vi "Main.vi"(8 "error in (no error)":errorcluster, 11 "ModuleAdmin":refnum<class "ModuleAdmin.lvclass">) -> ()   [LabVIEW 2014, in "SpecAnModule.lvlib"]
uses:
  SpecAnModule.lvlib
  <userlib>/NIST/ModuleAdminLib/ModuleAdmin/ModuleAdmin.lvclass
  SpecAnPlugins/SpecAnBaseClass/SpecAnBase.lvclass
  PublicAPI/Arguments/Requests/clStopArgument.ctl
  <userlib>/NIST/ModuleAdminLib/ModuleAdmin/ModuleAdmin.lvclass/ModuleAdmin.ctl
  <userlib>/NIST/BaseClasses/BasePlugin_class/BasePlugin.lvclass/BasePlugin.ctl
  <vilib>/Utility/error.llb/DialogType.ctl
  <userlib>/NIST/ModuleAdminLib/ModuleAdmin/Accessors/Read ShowPanel_.vi
  <userlib>/NIST/ModuleAdminLib/ModuleAdmin/Accessors/Write ShowPanel_.vi
  <userlib>/NIST/BaseClasses/BasePlugin_class/Accessors/Write PluginIniFilePath.vi
  <userlib>/NIST/BaseClasses/BasePlugin_class/Accessors/Read PluginIniFilePath.vi
  <userlib>/NIST/ModuleAdminLib/ModuleAdmin/Accessors/Read CloneRegRef.vi
  <vilib>/Utility/error.llb/Error Cluster From Error Code.vi
  <vilib>/ErrorRing/Error Ring.xnode
  <userlib>/NIST/ModuleAdminLib/CloneRegistration/CloneRegistration.lvclass
  <userlib>/NIST/BaseClasses/Object_class/BaseObject.lvclass
  <userlib>/NIST/ModuleAdminLib/ModuleAdmin.lvlib
panel:
  out "error out":errorcluster
  # "This is the template for your cloneable module.\nYou should modifiy this to perform the functionality\nthat you want it to perform"
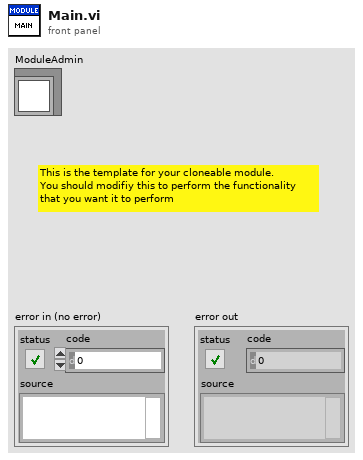
[diagram p1: front panel]
types:
  T1 = typedef "SpecAnModule.lvlib/clRequestEvents.ctl" = cluster{"StopRequest":refnum<user-event>, "PathToINI":refnum<user-event>, " LoadPlugin":refnum<user-event>, "ShowPanel":refnum<user-event>, "PrefDlg":refnum<user-event>, "Initialize":refnum<user-event>, "Close":refnum<user-event>, "Abort":refnum<user-event>, "Fetch":refnum<user-event>, "Read":refnum<user-event>, "Configure":refnum<user-event>, "GetTraceName":refnum<user-event>, "Initiate":refnum<user-event>}
  T2 = typedef "SpecAnModule.lvlib/clBroadcastEvents.ctl" = cluster{"DidInit":refnum<user-event>, "StatusUpdate":refnum<user-event>, "ErrorReport":refnum<user-event>, "DidStop":refnum<user-event>, "PathToINI":refnum<user-event>, "TraceName":refnum<user-event>}
  T3 = typedef "SpecAnModule.lvlib/clStopArgument.ctl" = cluster{"Exit via Stop Module Req?":bool, "Wait for Module to stop?":bool, "ModuleAdmin":refnum<class "ModuleAdmin.lvclass">}
  T4 = enum32{"Invalid", "Standard", "Closed", "Hidden", "Minimized", "Maximized"}
  T5 = typedef "DialogType.ctl" = u16
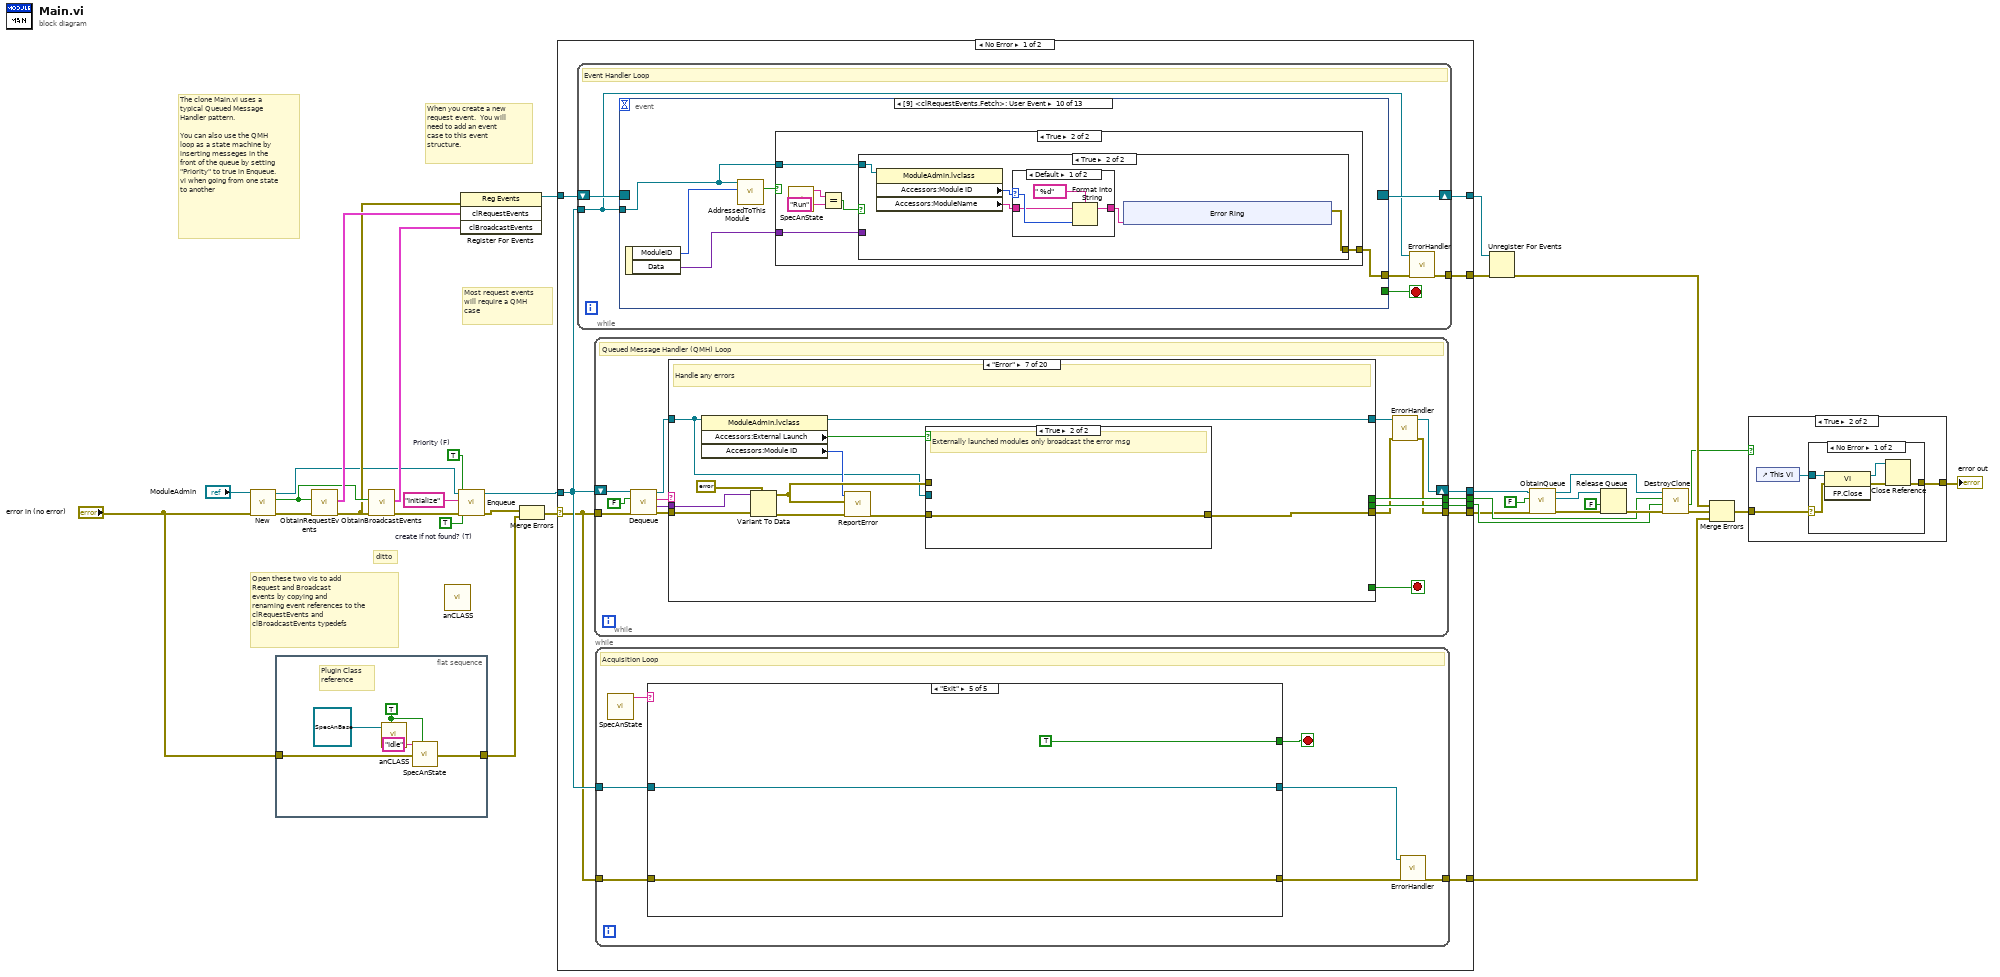
[diagram p0: block diagram]
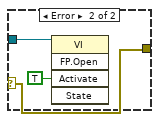
[diagram p3: hidden frame]
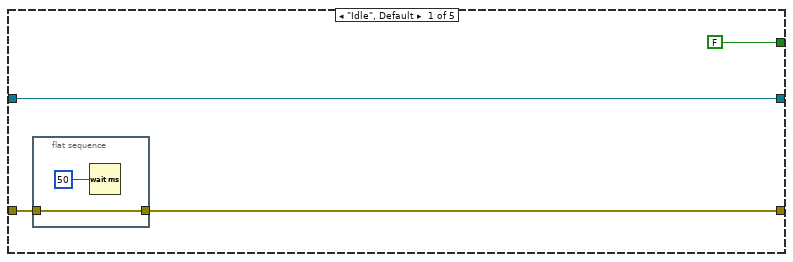
[diagram p4: hidden frame]
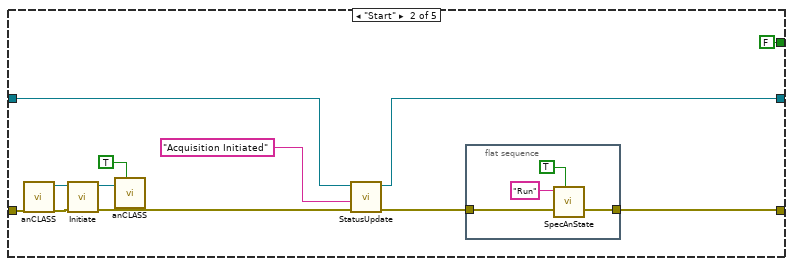
[diagram p5: hidden frame]
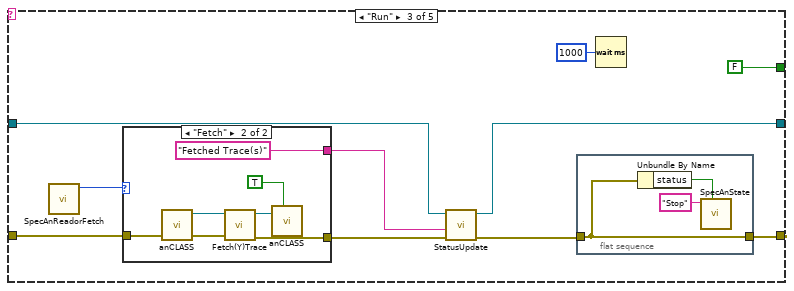
[diagram p6: hidden frame]
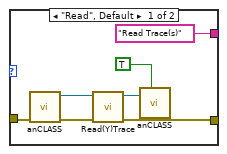
[diagram p7: hidden frame]
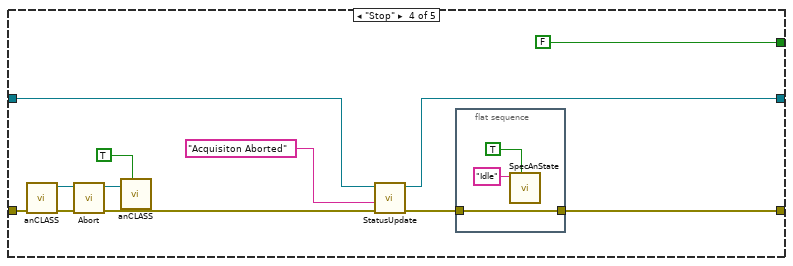
[diagram p8: hidden frame]
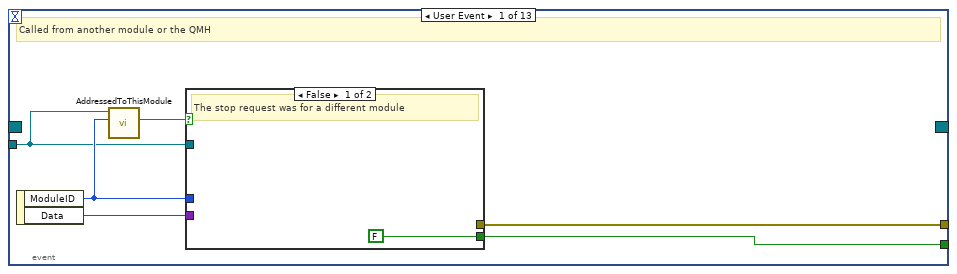
[diagram p9: hidden frame]
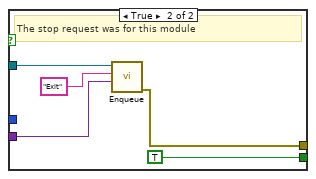
[diagram p10: hidden frame]
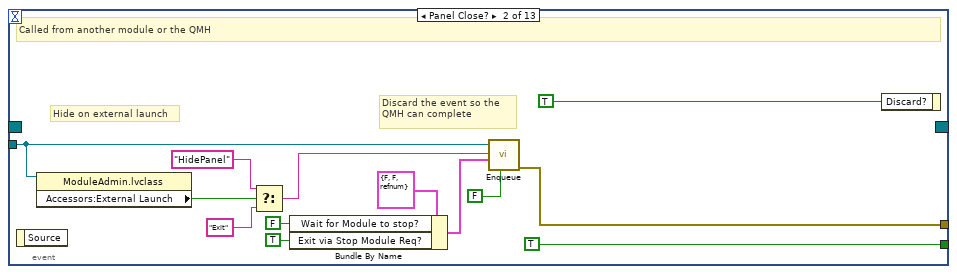
[diagram p11: hidden frame]
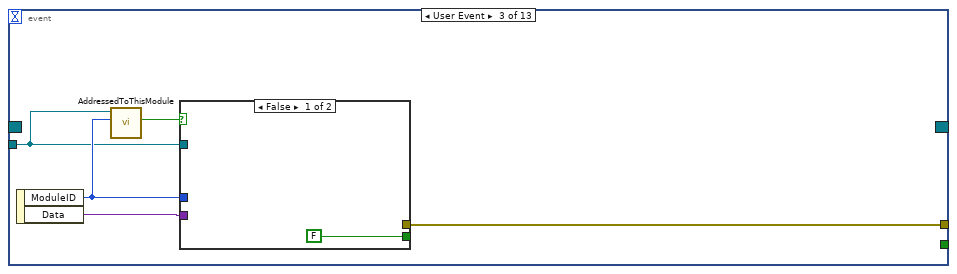
[diagram p12: hidden frame]
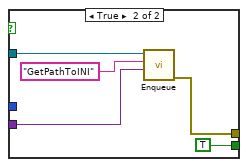
[diagram p13: hidden frame]
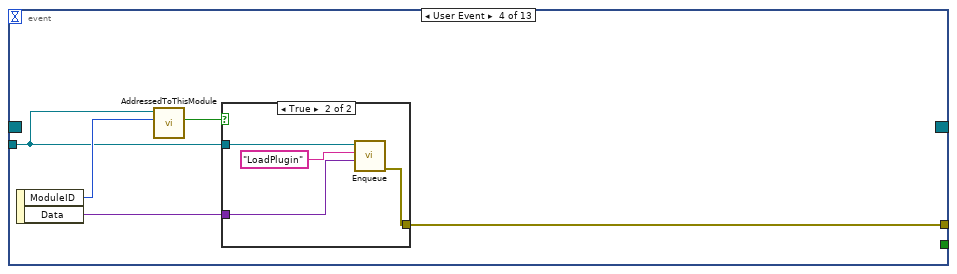
[diagram p14: hidden frame]
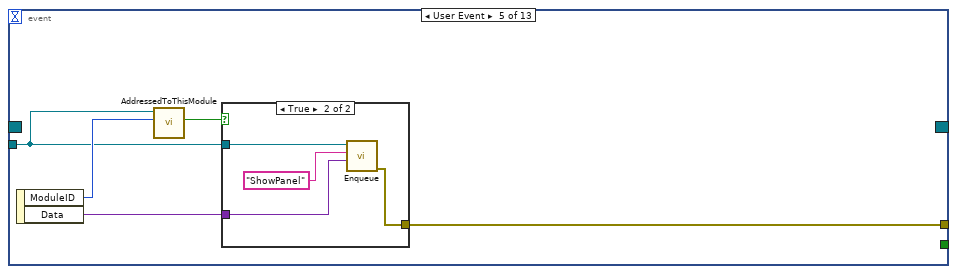
[diagram p16: hidden frame]
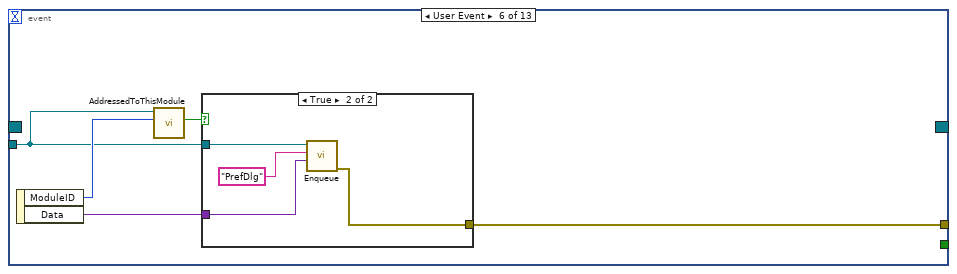
[diagram p18: hidden frame]
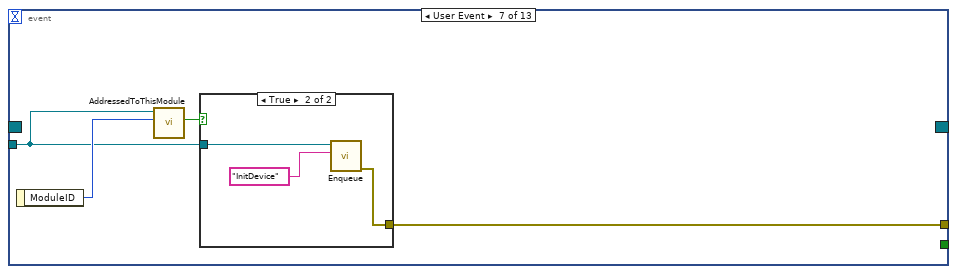
[diagram p20: hidden frame]
diagram:
  w17 = TRUE  # create if not found? (T)
  w18 = TRUE  # Priority (F)
  # "The clone Main.vi uses a typical Queued Message Handler pattern.  \n\nYou can also use the QMH loop as a state machine by inserting messeges in the front of the queue by setting \"Priority\" to true in Enqueue.vi when going from one state to another"
  # "Open these two vis to add\nRequest and Broadcast \nevents by copying and \nrenaming event references to the \nclRequestEvents and \nclBroadcastEvents typedefs"
  # "ditto"
  # "Most request events\nwill require a QMH\ncase"
  # "When you create a new request event.  You will need to add an event case to this event structure."
  n1 = call <userlib>:"New.vi"("error in (no error)"="error in (no error)", "ModuleAdmin"="ModuleAdmin") -> ("error out"=w25:errorcluster, "First?"=w33:bool, "ModuleAdmin"=w23:refnum<class "ModuleAdmin.lvclass">)  [unwired: 6 in, 1 out]
  n2 = flat-sequence {
    tunnel: "error in (no error)" -> [w38]
    tunnel: [w38] -> w13
    frame #0 {
      w36 = TRUE ("Set? (f)")
      # "Plugin Class\nreference"
      n3 = call "anCLASS.vi"("Set? (f)"=w36, "SpecAnPlugins.lvlib In"=refnum<class "SpecAnBase.lvclass"> refnum ("MyPlugins.lvlib:MyPluginsBase.lvclass")) -> ()  [unwired: 9 in, 1 out]
      n4 = call "SpecAnState.vi"("Set Boolean"=w36, "State In"="Idle") -> ()  [unwired: 9 in, 1 out]
    }
  }
  n5 = call "ObtainRequestEvents.vi"("error in (no error)"=w25, "CreateNew (F)"=w33) -> ("error out"=w32:errorcluster, "clRequestEvents"=w34:T1)  [unwired: 8 in]
  n6 = call "ObtainBroadcastEvents.vi"("error in (no error)"=w32, "CreateNew? (F)"=w33) -> ("error out"=w24:errorcluster, "clBroadcastEvents"=w31:T2)  [unwired: 8 in]
  n7 = call "anCLASS.vi"() -> ()  [unwired: 11 in, 1 out]
  n8 = call "Enqueue.vi"("create if not found? (T)"=w17, "Priority (F)"=w18, "error in (no error)"=w24, "Message"="Initialize", "ModuleAdmin"=w23) -> ("error out"=w14:errorcluster, "ModuleAdmin Out"=w22:refnum<class "ModuleAdmin.lvclass">)  [unwired: 5 in]
  n9 = register-events(error in=w32, w34, w31) -> (reference out=w30:refnum<event-registration>)  [unwired: 1 in, 1 out]
  n10 = Merge Errors(w14, w13) -> (w15:errorcluster)
  n11 = case shown="No Error" w15 {
    selector: w15 -> [w40 w604]
    tunnel: w22 -> [w41 w598]
    tunnel: [w43 w597] -> w3
    tunnel: w30 -> [w49 w599]
    tunnel: [w48 w602] -> w4
    tunnel: [w47 _] -> w7
    tunnel: [w46 _] -> w6
    tunnel: [w45 w597] -> w29
    tunnel: [w44 w599] -> w28
    tunnel: [w42 w597] -> w1
    frame No Error {
      n12 = while {
        tunnel: w41 -> [w119]
        shift-right: [w122] -> w44
        shift-left: w49 -> [w123]
        tunnel: [w120] -> w45
        stop <- w124 stop-if-true
        # "Event Handler Loop"
        n13 = event shown="[9] <clRequestEvents.Fetch>: User Event" {
          selector: w123 -> [_ _ _ _ _ _ _ _ _ _ _ _ _]
          dyn-events: [_ _ _ _ _ _ _ _ _ _ _ _ _] -> w122
          timeout: _ -> [_ _ _ _ _ _ _ _ _ _ _ _ _]
          tunnel: w119 -> [w125 w138 w150 w161 w170 w179 w188 w195 w217 w224 w257 w264 w271]
          tunnel: [w128 TRUE _ _ _ _ _ _ _ _ _ _ _] -> w124
          tunnel: [w127 w148 w151 w163 w172 w181 w189 w196 w218 w225 w258 w265 w272] -> w121
          event User Event {
            # "Called from another module or the QMH"
            n14 = event-data() -> ("ModuleID"=w129:i32, "Data"=w126:variant)  [unwired: 1 in]
            n15 = call <userlib>:"AddressedToThisModule.vi"("ModuleID"=w129, "ModuleAdmin"=w125) -> ("AddressedToThisInstance?"=w130:bool)  [unwired: 8 in, 1 out]
            n16 = case shown="False" w130 {
              tunnel: w129 -> [_ _]
              tunnel: w125 -> [_ w136]
              tunnel: [FALSE TRUE] -> w128
              tunnel: [_ w134] -> w127
              tunnel: w126 -> [_ w132]
              frame False {
                # "The stop request was for a different module"
              }
              frame True {
                # "The stop request was for this module"
                n17 = call "Enqueue.vi"("Message Data"=w132, "Message"="Exit", "ModuleAdmin"=w136) -> ("error out"=w134:errorcluster)  [unwired: 7 in, 1 out]
              }
            }
          }
          event Panel Close? {
            # "Hide on external launch"
            # "Discard the event so the QMH can complete"
            # "Called from another module or the QMH"
            n18 = event-data() -> ()  [unwired: 1 in, 1 out]
            n19 = property class="ModuleAdmin.lvclass"(reference=w138) -> ("Accessors:External Launch"=w140:bool)  [unwired: 1 in, 2 out]
            n20 = Select(t="HidePanel", s=w140, f="Exit" ("Message")) -> (s? t:f=w142:string)
            n21 = Bundle By Name(cluster=T3 {"Exit via Stop Module Req?"=FALSE, "Wait for Module to stop?"=FALSE, "ModuleAdmin"=refnum} ("Stop Argument"), "Wait for Module to stop?"=FALSE, "Exit via Stop Module Req?"=TRUE) -> (w145:T3)
            n22 = call "Enqueue.vi"("create if not found? (T)"=FALSE, "Message Data"=w145, "Message"=w142, "ModuleAdmin"=w138) -> ("error out"=w148:errorcluster)  [unwired: 6 in, 1 out]
            n23 = event-data("Discard?"=TRUE) -> ()  [unwired: 1 in, 1 out]
          }
          event User Event {
            n24 = event-data() -> ("ModuleID"=w152:i32, "Data"=w153:variant)  [unwired: 1 in]
            n25 = call <userlib>:"AddressedToThisModule.vi"("ModuleID"=w152, "ModuleAdmin"=w150) -> ("AddressedToThisInstance?"=w154:bool)  [unwired: 8 in, 1 out]
            n26 = case shown="False" w154 {
              tunnel: w152 -> [_ _]
              tunnel: w150 -> [_ w160]
              tunnel: [FALSE TRUE] -> _
              tunnel: [_ w158] -> w151
              tunnel: w153 -> [_ w156]
              frame False {
                # "The stop request was for a different module"
              }
              frame True {
                # "The stop request was for this module"
                n27 = call "Enqueue.vi"("Message Data"=w156, "Message"="GetPathToINI", "ModuleAdmin"=w160) -> ("error out"=w158:errorcluster)  [unwired: 7 in, 1 out]
              }
            }
          }
          event User Event {
            n28 = event-data() -> ("ModuleID"=w165:i32, "Data"=w162:variant)  [unwired: 1 in]
            n29 = call <userlib>:"AddressedToThisModule.vi"("ModuleID"=w165, "ModuleAdmin"=w161) -> ("AddressedToThisInstance?"=w164:bool)  [unwired: 8 in, 1 out]
            n30 = case shown="True" w164 {
              tunnel: [_ w166] -> w163
              tunnel: w161 -> [_ w169]
              tunnel: w162 -> [_ w167]
              frame False {
              }
              frame True {
                n31 = call "Enqueue.vi"("Message Data"=w167, "Message"="LoadPlugin", "ModuleAdmin"=w169) -> ("error out"=w166:errorcluster)  [unwired: 7 in, 1 out]
              }
            }
          }
          event User Event {
            n32 = event-data() -> ("ModuleID"=w174:i32, "Data"=w171:variant)  [unwired: 1 in]
            n33 = call <userlib>:"AddressedToThisModule.vi"("ModuleID"=w174, "ModuleAdmin"=w170) -> ("AddressedToThisInstance?"=w173:bool)  [unwired: 8 in, 1 out]
            n34 = case shown="True" w173 {
              tunnel: [_ w175] -> w172
              tunnel: w170 -> [_ w178]
              tunnel: w171 -> [_ w176]
              frame False {
              }
              frame True {
                n35 = call "Enqueue.vi"("Message Data"=w176, "Message"="ShowPanel", "ModuleAdmin"=w178) -> ("error out"=w175:errorcluster)  [unwired: 7 in, 1 out]
              }
            }
          }
          event User Event {
            n36 = event-data() -> ("ModuleID"=w183:i32, "Data"=w180:variant)  [unwired: 1 in]
            n37 = call <userlib>:"AddressedToThisModule.vi"("ModuleID"=w183, "ModuleAdmin"=w179) -> ("AddressedToThisInstance?"=w182:bool)  [unwired: 8 in, 1 out]
            n38 = case shown="True" w182 {
              tunnel: [_ w184] -> w181
              tunnel: w179 -> [_ w187]
              tunnel: w180 -> [_ w185]
              frame False {
              }
              frame True {
                n39 = call "Enqueue.vi"("Message Data"=w185, "Message"="PrefDlg", "ModuleAdmin"=w187) -> ("error out"=w184:errorcluster)  [unwired: 7 in, 1 out]
              }
            }
          }
          event User Event {
            n40 = event-data() -> ("ModuleID"=w191:i32)  [unwired: 1 in]
            n41 = call <userlib>:"AddressedToThisModule.vi"("ModuleID"=w191, "ModuleAdmin"=w188) -> ("AddressedToThisInstance?"=w190:bool)  [unwired: 8 in, 1 out]
            n42 = case shown="True" w190 {
              tunnel: [_ w192] -> w189
              tunnel: w188 -> [_ w194]
              frame False {
              }
              frame True {
                n43 = call "Enqueue.vi"("Message"="InitDevice", "ModuleAdmin"=w194) -> ("error out"=w192:errorcluster)  [unwired: 8 in, 1 out]
              }
            }
          }
          event User Event {
            n44 = event-data() -> ("ModuleID"=w198:i32)  [unwired: 1 in]
            n45 = call <userlib>:"AddressedToThisModule.vi"("ModuleID"=w198, "ModuleAdmin"=w195) -> ("AddressedToThisInstance?"=w197:bool)  [unwired: 8 in, 1 out]
            n46 = case shown="True" w197 {
              tunnel: [_ w204] -> w196
              tunnel: w195 -> [_ w216]
              frame False {
              }
              frame True {
                n47 = call "Enqueue.vi"("Message"="ConfigureAcq", "ModuleAdmin"=w216) -> ("error out"=w214:errorcluster, "ModuleAdmin Out"=w212:refnum<class "ModuleAdmin.lvclass">)  [unwired: 8 in]
                n48 = call "Enqueue.vi"("error in (no error)"=w214, "Message"="ConfigureFreq", "ModuleAdmin"=w212) -> ("error out"=w203:errorcluster, "ModuleAdmin Out"=w202:refnum<class "ModuleAdmin.lvclass">)  [unwired: 7 in]
                n49 = call "Enqueue.vi"("error in (no error)"=w203, "Message"="ConfigureLvl", "ModuleAdmin"=w202) -> ("error out"=w200:errorcluster, "ModuleAdmin Out"=w201:refnum<class "ModuleAdmin.lvclass">)  [unwired: 7 in]
                n50 = call "Enqueue.vi"("error in (no error)"=w200, "Message"="ConfigureSwCo", "ModuleAdmin"=w201) -> ("error out"=w211:errorcluster, "ModuleAdmin Out"=w210:refnum<class "ModuleAdmin.lvclass">)  [unwired: 7 in]
                n51 = call "Enqueue.vi"("error in (no error)"=w211, "Message"="ConfigureTraceType", "ModuleAdmin"=w210) -> ("error out"=w208:errorcluster, "ModuleAdmin Out"=w207:refnum<class "ModuleAdmin.lvclass">)  [unwired: 7 in]
                n52 = call "Enqueue.vi"("error in (no error)"=w208, "Message"="ConfigureTrigger", "ModuleAdmin"=w207) -> ("error out"=w204:errorcluster)  [unwired: 7 in, 1 out]
              }
            }
          }
          event User Event {
            n53 = event-data() -> ("ModuleID"=w220:i32)  [unwired: 1 in]
            n54 = call <userlib>:"AddressedToThisModule.vi"("ModuleID"=w220, "ModuleAdmin"=w217) -> ("AddressedToThisInstance?"=w219:bool)  [unwired: 8 in, 1 out]
            n55 = case shown="True" w219 {
              tunnel: [_ w221] -> w218
              tunnel: w217 -> [_ w223]
              frame False {
              }
              frame True {
                n56 = call "Enqueue.vi"("Message"="InitAcq", "ModuleAdmin"=w223) -> ("error out"=w221:errorcluster)  [unwired: 8 in, 1 out]
              }
            }
          }
          event User Event {
            n57 = event-data() -> ("ModuleID"=w228:i32, "Data"=w226:variant)  [unwired: 1 in]
            n58 = call <userlib>:"AddressedToThisModule.vi"("ModuleID"=w228, "ModuleAdmin"=w224) -> ("AddressedToThisInstance?"=w227:bool)  [unwired: 8 in, 1 out]
            n59 = case shown="True" w227 {
              tunnel: w226 -> [_ w234]
              tunnel: [_ w233] -> w225
              tunnel: w224 -> [_ w229]
              frame False {
              }
              frame True {
                n60 = call "SpecAnState.vi"() -> ("State Out"=w231:string)  [unwired: 11 in]
                n61 = Equal?(x=w231, y="Run") -> (x = y?=w230:bool)
                n62 = case shown="True" w230 {
                  tunnel: w234 -> [w239 _]
                  tunnel: [w238 w241] -> w233
                  tunnel: w229 -> [_ w244]
                  frame False {
                    n63 = Variant To Data(type=enum16{"Read", "Fetch"}."Read" ("enumFetchorRead 2"), Variant=w239) -> (data=w236:enum16{"Read", "Fetch"}, error out=w238:errorcluster)  [unwired: 1 in]
                    n64 = call "SpecAnReadorFetch.vi"("Set Boolean"=TRUE, "enumFetchorRead"=w236) -> ()  [unwired: 9 in, 1 out]
                  }
                  frame True {
                    n65 = property class="ModuleAdmin.lvclass"(reference=w244) -> ("Accessors:Module ID"=w243:i32, "Accessors:ModuleName"=w242:string)  [unwired: 1 in, 2 out]
                    n66 = case shown="Default" w243 {
                      selector: w243 -> [w255 _]
                      tunnel: [w253 w256] -> w240
                      tunnel: w242 -> [w254 w256]
                      frame Default {
                        n67 = Format Into String(format string=" %d", initial string=w254, w255) -> (resulting string=w253:string)  [unwired: 1 in, 1 out]
                      }
                      frame ..-1 {
                      }
                    }
                    n68 = xnode "Error Ring"("parameter 0"=w240) -> ("error out"=w241:errorcluster)
                  }
                }
              }
            }
          }
          event User Event {
            n69 = event-data() -> ("ModuleID"=w260:i32)  [unwired: 1 in]
            n70 = call <userlib>:"AddressedToThisModule.vi"("ModuleID"=w260, "ModuleAdmin"=w257) -> ("AddressedToThisInstance?"=w259:bool)  [unwired: 8 in, 1 out]
            n71 = case shown="True" w259 {
              tunnel: [_ w261] -> w258
              tunnel: w257 -> [_ w263]
              frame False {
              }
              frame True {
                n72 = call "Enqueue.vi"("Message"="GetTraceName", "ModuleAdmin"=w263) -> ("error out"=w261:errorcluster)  [unwired: 8 in, 1 out]
              }
            }
          }
          event User Event {
            n73 = event-data() -> ("ModuleID"=w267:i32)  [unwired: 1 in]
            n74 = call <userlib>:"AddressedToThisModule.vi"("ModuleID"=w267, "ModuleAdmin"=w264) -> ("AddressedToThisInstance?"=w266:bool)  [unwired: 8 in, 1 out]
            n75 = case shown="True" w266 {
              tunnel: [_ w268] -> w265
              tunnel: w264 -> [_ w270]
              frame False {
              }
              frame True {
                n76 = call "Enqueue.vi"("Message"="CloseDevice", "ModuleAdmin"=w270) -> ("error out"=w268:errorcluster)  [unwired: 8 in, 1 out]
              }
            }
          }
          event User Event {
            n77 = event-data() -> ("ModuleID"=w274:i32)  [unwired: 1 in]
            n78 = call <userlib>:"AddressedToThisModule.vi"("ModuleID"=w274, "ModuleAdmin"=w271) -> ("AddressedToThisInstance?"=w273:bool)  [unwired: 8 in, 1 out]
            n79 = case shown="True" w273 {
              tunnel: [_ w275] -> w272
              tunnel: w271 -> [_ w277]
              frame False {
              }
              frame True {
                n80 = call "Enqueue.vi"("Message"="Abort", "ModuleAdmin"=w277) -> ("error out"=w275:errorcluster)  [unwired: 8 in, 1 out]
              }
            }
          }
        }
        n81 = call "ErrorHandler.vi"("error in (no error)"=w121, "ModuleAdmin"=w119) -> ("error out"=w120:errorcluster)  [unwired: 8 in, 1 out]
      }
      n82 = while {
        tunnel: w40 -> [w290]
        tunnel: [w284] -> w43
        tunnel: [w286] -> w47
        tunnel: [w285] -> w46
        shift-right: [w281] -> w48
        shift-left: w41 -> [w280]
        stop <- w291 stop-if-true
        # "Queued Message Handler (QMH) Loop"
        n83 = call "Dequeue.vi"("error in (no error)"=w290, "create if not found? (f)"=FALSE ("create if not found? (T)"), "ModuleAdmin"=w280) -> ("error out"=w289:errorcluster, "Message Data"=w287:variant, "Message"=w288:string, "ModuleAdmin Out"=w279:refnum<class "ModuleAdmin.lvclass">)  [unwired: 5 in]
        n84 = case shown="\"Error\"" w288 {
          selector: w288 -> [_ _ _ _ _ _ _ _ w428 w440 _ _ _ _ _ _ w539 _ _ _]
          tunnel: [_ _ _ _ _ TRUE _ TRUE _ _ _ _ _ _ _ _ _ _ _ _] -> w291
          tunnel: w279 -> [w312 w328 w334 w382 w392 w395 w404 w421 w431 w441 w484 w493 w503 w513 w523 w533 w538 w572 w589 w591]
          tunnel: [w301 w321 w335 w383 w388 w401 w405 w423 w427 w447 w485 w494 w504 w514 w524 w534 w537 w579 w590 w592] -> w283
          tunnel: w289 -> [w294 w331 w344 w380 w390 w400 w413 _ _ w443 w480 w495 w505 w515 w525 w535 w541 w580 w585 w593]
          tunnel: w287 -> [_ w330 w346 _ _ w399 w412 _ _ _ _ _ _ _ _ _ _ _ _ _]
          tunnel: [_ _ _ _ _ w397 _ _ _ _ _ _ _ _ _ _ _ _ _ _] -> w286
          tunnel: [_ _ _ _ _ w396 _ _ _ _ _ _ _ _ _ _ _ _ _ _] -> w285
          tunnel: [w295 w327 w332 w378 w392 w395 w403 w421 w425 w446 w483 w492 w502 w512 w522 w532 w536 w578 w588 w591] -> w282
          frame "Initialize" {
            # "Initialize is always called after ObtainQueue.vi is run"
            n85 = property class="ModuleAdmin.lvclass"(reference=w312, error in=w294) -> (reference out=w299:refnum<class "ModuleAdmin.lvclass">, error out=w309:errorcluster, "Accessors:ShowPanel_"=w298:bool, "Accessors:External Launch"=w297:bool, "Accessors:Module ID"=w292:i32, "Accessors:ModuleName"=w293:string)
            n86 = Compound Arithmetic op=OR(w298, invert w297) -> (w296:bool)
            n87 = Select(t=T4."Standard" ("Front Panel Window:State"), s=w296, f=T4."Hidden" ("Front Panel Window:State")) -> (s? t:f=w305:T4)
            n88 = invoke class="VI" method="FP.Open"(error in=w309, "State"=w305) -> (error out=w308:errorcluster)  [unwired: 3 in, 4 out]
            n89 = call <userlib>:"ModuleName.vi"("Name"=w293, "ModuleID"=w292) -> ("ModuleName"=w304:string)  [unwired: 9 in]
            n90 = property class="VI"(error in=w308, "Front Panel.Title"=w304) -> (reference out=w311:refnum<vi>, error out=w310:errorcluster)  [unwired: 1 in]
            n91 = invoke class="VI" method="FP.Center"(reference=w311, error in=w310) -> (error out=w300:errorcluster)  [unwired: 1 in, 2 out]
            n92 = case shown="True" w297 {
              tunnel: [w313 w319] -> w302
              tunnel: [w314 w316] -> w295
              tunnel: w300 -> [w313 w318]
              tunnel: w299 -> [w314 w315]
              frame False {
              }
              frame True {
                n93 = call <userlib>:"WaitOnModuleSync.vi"("error in (no error)"=w318, "ModuleAdmin"=w315) -> ("error out"=w320:errorcluster, "ModuleAdmin"=w317:refnum<class "ModuleAdmin.lvclass">)  [unwired: 8 in]
                n94 = call <userlib>:"WaitOnEventSync.vi"("error in (no error)"=w320, "ModuleAdmin"=w317) -> ("error out"=w319:errorcluster, "ModuleAdmin"=w316:refnum<class "ModuleAdmin.lvclass">)  [unwired: 8 in]
              }
            }
            n95 = call "DidInit.vi"("Init?"=TRUE, "error in (no error)"=w302, "ModuleAdmin"=w295) -> ("error out"=w301:errorcluster)  [unwired: 8 in]
          }
          frame "ShowPanel" {
            # "The frontpanel can be shown or hidden"
            n96 = Variant To Data(error in=w331, type=TRUE, Variant=w330) -> (data=w323:bool, error out=w326:errorcluster)
            n97 = property class="ModuleAdmin.lvclass"(reference=w328, "Accessors:ShowPanel_"=w323) -> (reference out=w327:refnum<class "ModuleAdmin.lvclass">)  [unwired: 1 in, 1 out]
            n98 = Select(t=T4."Standard" ("Front Panel Window:State"), s=w323, f=T4."Hidden" ("Front Panel Window:State")) -> (s? t:f=w322:T4)
            n99 = property class="VI"(error in=w326, "FP.State"=w322) -> (error out=w321:errorcluster)  [unwired: 1 in, 1 out]
          }
          frame "LoadPlugin" {
            # "Dynamically loads and initializes a plugin from the .ini file"
            n100 = Variant To Data(error in=w344, type=path "", Variant=w346) -> (data=w333:path, error out=w343:errorcluster)
            n101 = call <userlib>:"GetPathToClass.vi"("error in (no error)"=w343, "configuration file path"=w333) -> ("error IO"=w339:errorcluster, "PathToClass"=w342:path)  [unwired: 8 in]
            n102 = Current VI's Path() -> (path=w341:path)
            n103 = Build Path(base path=w341, name or relative path=w342) -> (appended path=w340:path)
            n104 = call <vilib>:"Check if File or Folder Exists.vi"("error in (no error)"=w339, "path"=w340) -> ("error out"=w336:errorcluster, "file or folder exists?"=w338:bool, "dup path"=w337:path)  [unwired: 7 in]
            n105 = case shown="True" w338 {
              selector: w338 -> [_ w360]
              tunnel: w337 -> [w349 w371]
              tunnel: w336 -> [_ w361]
              tunnel: [w348 w373] -> w335
              tunnel: w334 -> [w347 w368]
              tunnel: w333 -> [_ w369]
              tunnel: [w347 w367] -> w332
              frame False {
                n106 = Path To String(path=w349) -> (string=w350:string)
                n107 = xnode "Error Ring"("parameter 0"=w350) -> ("error out"=w348:errorcluster)
              }
              frame True {
                n108 = call "anCLASS.vi"() -> ("SpecAnPlugins.lvlib Out"=w359:refnum<class "SpecAnBase.lvclass">)  [unwired: 11 in]
                n109 = call "CheckOnIdle.vi"("error in (no error)"=w361, "ChangeOccured? (F)"=w360, "SpecAnPlugins.lvlib In"=w359) -> ("Error Out"=w358:errorcluster)  [unwired: 7 in, 1 out]
                n110 = call-dynamic "LoadClassFromFile.vi"("error in (no error)"=w358, "class path"=w371, "reference in"=w359) -> ("error out"=w370:errorcluster, "reference out"=w372:refnum<class "SpecAnBase.lvclass">)  [unwired: 7 in]
                n111 = Path To String(path=w371) -> (string=w375:string)
                n112 = Format Into String(format string="Plugin %s loaded ", w375) -> (resulting string=w374:string)  [unwired: 2 in, 1 out]
                n113 = property class="SpecAnBase.lvclass"(reference=w372, error in=w370, "Accessors:PluginIniFilePath"=w369) -> (reference out=w366:refnum<class "SpecAnBase.lvclass">, error out=w365:errorcluster)
                n114 = call-dynamic "DefaultFromIni.vi"("error in (no error)"=w365, "SpecAnPlugins.lvlib"=w366) -> ("error out"=w364:errorcluster, "SpecAnPlugins.lvlib"=w363:refnum<class "SpecAnBase.lvclass">)  [unwired: 8 in]
                n115 = call "anCLASS.vi"("Set? (f)"=TRUE, "SpecAnPlugins.lvlib In"=w363) -> ()  [unwired: 9 in, 1 out]
                n116 = call "StatusUpdate.vi"("error in (no error)"=w364, "Status"=w374, "Module"=w368) -> ("error out"=w373:errorcluster, "Module"=w367:refnum<class "ModuleAdmin.lvclass">)  [unwired: 7 in]
              }
            }
          }
          frame "GetPathToINI" {
            # "Broadcast the path to the .ini file"
            n117 = call "anCLASS.vi"() -> ("SpecAnPlugins.lvlib Out"=w377:refnum<class "SpecAnBase.lvclass">)  [unwired: 11 in]
            n118 = property class="SpecAnBase.lvclass"(reference=w377, error in=w380) -> (error out=w379:errorcluster, "Accessors:PluginIniFilePath"=w381:path)  [unwired: 1 out]
            n119 = property class="ModuleAdmin.lvclass"(reference=w382) -> (reference out=w378:refnum<class "ModuleAdmin.lvclass">, "Accessors:Module ID"=w384:i32)  [unwired: 1 in, 1 out]
            n120 = call "PathToINIBroadcast.vi"("error in (no error)"=w379, "PathToINI"=w381, "ModuleID"=w384) -> ("error out"=w383:errorcluster)  [unwired: 8 in]
          }
          frame "PrefDlg" {
            # "Launch the modal Preferences dialog"
            n121 = call "anCLASS.vi"() -> ("SpecAnPlugins.lvlib Out"=w391:refnum<class "SpecAnBase.lvclass">)  [unwired: 11 in]
            n122 = call-dynamic "PrefDialog.vi"("error in (no error)"=w390, "SpecAnPlugins.lvlib"=w391) -> ("error out"=w389:errorcluster, "Change Occured?"=w386:bool, "SpecAnPlugins.lvlib"=w387:refnum<class "SpecAnBase.lvclass">)  [unwired: 7 in]
            n123 = call "CheckOnIdle.vi"("OverwriteClass? (F)"=TRUE, "error in (no error)"=w389, "ChangeOccured? (F)"=w386, "SpecAnPlugins.lvlib In"=w387) -> ("Error Out"=w388:errorcluster)  [unwired: 6 in, 1 out]
          }
          frame "Exit" {
            # "Called by the StopRequest event handler case"
            n124 = control-ref of="This VI"() -> (w398:refnum<vi>)
            n125 = call "HandleExit.vi"("error in (no error)"=w400, "VI Refnum"=w398, "StopArgument"=w399, "ModuleAdmin"=w395) -> ("error out"=w401:errorcluster, "Exit via Stop Module Req?"=w396:bool, "WaitForStop?"=w397:bool)  [unwired: 5 in]
            n126 = call "SpecAnState.vi"("Set Boolean"=TRUE, "State In"="Exit") -> ()  [unwired: 9 in, 1 out]
          }
          frame "Error" {
            # "Handle any errors"
            n127 = property class="ModuleAdmin.lvclass"(reference=w404) -> (reference out=w403:refnum<class "ModuleAdmin.lvclass">, "Accessors:External Launch"=w408:bool, "Accessors:Module ID"=w406:i32)  [unwired: 1 in, 1 out]
            n128 = Variant To Data(error in=w413, type=errorcluster {"status"=FALSE, "code"=0, "source"=""} ("error constant"), Variant=w412) -> (data=w407:errorcluster, error out=w410:errorcluster)
            n129 = call "ReportError.vi"("error in (no error)"=w410, "ErrorReported"=w407, "ModuleID"=w406) -> ("error out"=w409:errorcluster)  [unwired: 8 in]
            n130 = case shown="True" w408 {
              tunnel: w409 -> [w417 w418]
              tunnel: w407 -> [w416 _]
              tunnel: [w415 w418] -> w405
              tunnel: w404 -> [w414 _]
              frame False {
                # "Todo:  Add an event to ask the user\nIf the module should stop or continue"
                # "Stand alone: now, force an exit"
                n131 = call <vilib>:"Simple Error Handler.vi"("error in (no error)"=w416) -> ()  [unwired: 4 in, 5 out]
                n132 = call "StopRequest.vi"("error in (no error)"=w417, "ModuleAdmin"=w414) -> ("error out"=w415:errorcluster)  [unwired: 8 in, 1 out]
              }
              frame True {
                # "Externally launched modules only broadcast the error msg"
              }
            }
          }
          frame "QueueError" {
            n133 = call "StatusUpdate.vi"("Status"=" Queue Error" ("format string"), "Module"=w421) -> ("error out"=w424:errorcluster, "Module"=w422:refnum<class "ModuleAdmin.lvclass">)  [unwired: 8 in]
            n134 = call "StopRequest.vi"("error in (no error)"=w424, "ModuleAdmin"=w422) -> ("error out"=w423:errorcluster)  [unwired: 8 in, 1 out]
          }
          frame Default {
            # "Called only if a message was queued and no QMH case was created"
            n135 = property class="ModuleAdmin.lvclass"(reference=w431) -> (reference out=w425:refnum<class "ModuleAdmin.lvclass">, "Accessors:Module ID"=w430:i32, "Accessors:ModuleName"=w426:string)  [unwired: 1 in, 1 out]
            n136 = call <userlib>:"ModuleName.vi"("Name"=w426, "ModuleID"=w430) -> ("ModuleName"=w429:string)  [unwired: 9 in]
            n137 = xnode "Error Ring"("parameter 0"=w428, "parameter 1"=w429) -> ("error out"=w427:errorcluster)
          }
          frame "InitDevice" {
            n138 = call "SpecAnState.vi"() -> ("State Out"=w445:string)  [unwired: 11 in]
            n139 = Equal?(x=w445, y="Run") -> (x = y?=w442:bool)
            n140 = case shown="False" w442 {
              tunnel: [w455 w460] -> w447
              tunnel: [w454 w461] -> w446
              tunnel: w443 -> [w449 w462]
              tunnel: w441 -> [w448 w463]
              tunnel: w440 -> [_ _]
              frame False {
                n141 = call "anCLASS.vi"() -> ("SpecAnPlugins.lvlib Out"=w452:refnum<class "SpecAnBase.lvclass">)  [unwired: 11 in]
                n142 = call-dynamic "Initialize.vi"("error in (no error)"=w449, "SpecAnBase in"=w452) -> ("error out"=w456:errorcluster, "SpecAnBase out"=w450:refnum<class "SpecAnBase.lvclass">)  [unwired: 8 in]
                n143 = call "anCLASS.vi"("Set? (f)"=TRUE, "SpecAnPlugins.lvlib In"=w450) -> ()  [unwired: 9 in, 1 out]
                n144 = call "StatusUpdate.vi"("error in (no error)"=w456, "Status"="Device Initialized", "Module"=w448) -> ("error out"=w455:errorcluster, "Module"=w454:refnum<class "ModuleAdmin.lvclass">)  [unwired: 7 in]
              }
              frame True {
                n145 = property class="ModuleAdmin.lvclass"(reference=w463, error in=w462) -> (reference out=w461:refnum<class "ModuleAdmin.lvclass">, "Accessors:Module ID"=w458:i32, "Accessors:ModuleName"=w459:string)  [unwired: 1 out]
                n146 = case shown="Default" w458 {
                  selector: w458 -> [w467 _]
                  tunnel: [w465 w468] -> w457
                  tunnel: w459 -> [w466 w468]
                  frame Default {
                    n147 = Format Into String(format string=" %d", initial string=w466, w467) -> (resulting string=w465:string)  [unwired: 1 in, 1 out]
                  }
                  frame ..-1 {
                  }
                }
                n148 = xnode "Error Ring"("parameter 0"=w457) -> ("error out"=w460:errorcluster)
              }
            }
          }
          frame "ConfigureAcq" {
            w476 = TRUE ("ChangeOccured?")
            n149 = call "anCLASS.vi"() -> ("SpecAnPlugins.lvlib Out"=w481:refnum<class "SpecAnBase.lvclass">)  [unwired: 11 in]
            n150 = call-dynamic "ConfigureAcquisition.vi"("error in (no error)"=w480, "SpecAnBase in"=w481) -> ("error out"=w477:errorcluster, "SpecAnBase out"=w478:refnum<class "SpecAnBase.lvclass">)  [unwired: 8 in]
            n151 = call "CheckOnIdle.vi"("OverwriteClass? (F)"=w476, "error in (no error)"=w477, "ChangeOccured? (F)"=w476, "SpecAnPlugins.lvlib In"=w478) -> ("Error Out"=w479:errorcluster)  [unwired: 6 in, 1 out]
            n152 = call "StatusUpdate.vi"("error in (no error)"=w479, "Status"="Acquisition Configured", "Module"=w484) -> ("error out"=w485:errorcluster, "Module"=w483:refnum<class "ModuleAdmin.lvclass">)  [unwired: 7 in]
          }
          frame "ConfigureFreq" {
            w486 = TRUE ("Set? (f)")
            n153 = call "anCLASS.vi"() -> ("SpecAnPlugins.lvlib Out"=w490:refnum<class "SpecAnBase.lvclass">)  [unwired: 11 in]
            n154 = call-dynamic "ConfigureFrequency.vi"("error in (no error)"=w495, "SpecAnBase in"=w490) -> ("error out"=w488:errorcluster, "SpecAnBase out"=w489:refnum<class "SpecAnBase.lvclass">)  [unwired: 8 in]
            n155 = call "CheckOnIdle.vi"("OverwriteClass? (F)"=w486, "error in (no error)"=w488, "ChangeOccured? (F)"=w486, "SpecAnPlugins.lvlib In"=w489) -> ("Error Out"=w487:errorcluster)  [unwired: 6 in, 1 out]
            n156 = call "StatusUpdate.vi"("error in (no error)"=w487, "Status"="Frequency Configured", "Module"=w493) -> ("error out"=w494:errorcluster, "Module"=w492:refnum<class "ModuleAdmin.lvclass">)  [unwired: 7 in]
          }
          frame "ConfigureLvl" {
            w496 = TRUE ("Set? (f)")
            n157 = call "anCLASS.vi"() -> ("SpecAnPlugins.lvlib Out"=w500:refnum<class "SpecAnBase.lvclass">)  [unwired: 11 in]
            n158 = call-dynamic "ConfigureLevel.vi"("error in (no error)"=w505, "SpecAnBase in"=w500) -> ("error out"=w499:errorcluster, "SpecAnBase out"=w497:refnum<class "SpecAnBase.lvclass">)  [unwired: 8 in]
            n159 = call "CheckOnIdle.vi"("OverwriteClass? (F)"=w496, "error in (no error)"=w499, "ChangeOccured? (F)"=w496, "SpecAnPlugins.lvlib In"=w497) -> ("Error Out"=w498:errorcluster)  [unwired: 6 in, 1 out]
            n160 = call "StatusUpdate.vi"("error in (no error)"=w498, "Status"="Level Configured", "Module"=w503) -> ("error out"=w504:errorcluster, "Module"=w502:refnum<class "ModuleAdmin.lvclass">)  [unwired: 7 in]
          }
          frame "ConfigureSwCo" {
            w506 = TRUE ("Set? (f)")
            n161 = call "anCLASS.vi"() -> ("SpecAnPlugins.lvlib Out"=w510:refnum<class "SpecAnBase.lvclass">)  [unwired: 11 in]
            n162 = call-dynamic "ConfigureSweepCoupling.vi"("error in (no error)"=w515, "SpecAnBase in"=w510) -> ("error out"=w509:errorcluster, "SpecAnBase out"=w508:refnum<class "SpecAnBase.lvclass">)  [unwired: 8 in]
            n163 = call "CheckOnIdle.vi"("OverwriteClass? (F)"=w506, "error in (no error)"=w509, "ChangeOccured? (F)"=w506, "SpecAnPlugins.lvlib In"=w508) -> ("Error Out"=w507:errorcluster)  [unwired: 6 in, 1 out]
            n164 = call "StatusUpdate.vi"("error in (no error)"=w507, "Status"="SweepCoupling Configured", "Module"=w513) -> ("error out"=w514:errorcluster, "Module"=w512:refnum<class "ModuleAdmin.lvclass">)  [unwired: 7 in]
          }
          frame "ConfigureTraceType" {
            w516 = TRUE ("Set? (f)")
            n165 = call "anCLASS.vi"() -> ("SpecAnPlugins.lvlib Out"=w520:refnum<class "SpecAnBase.lvclass">)  [unwired: 11 in]
            n166 = call-dynamic "ConfigureTraceType.vi"("error in (no error)"=w525, "SpecAnBase in"=w520) -> ("error out"=w519:errorcluster, "SpecAnBase out"=w518:refnum<class "SpecAnBase.lvclass">)  [unwired: 8 in]
            n167 = call "CheckOnIdle.vi"("OverwriteClass? (F)"=w516, "error in (no error)"=w519, "ChangeOccured? (F)"=w516, "SpecAnPlugins.lvlib In"=w518) -> ("Error Out"=w517:errorcluster)  [unwired: 6 in, 1 out]
            n168 = call "StatusUpdate.vi"("error in (no error)"=w517, "Status"="TraceType Configured", "Module"=w523) -> ("error out"=w524:errorcluster, "Module"=w522:refnum<class "ModuleAdmin.lvclass">)  [unwired: 7 in]
          }
          frame "ConfigureTrigger" {
            w526 = TRUE ("Set? (f)")
            n169 = call "anCLASS.vi"() -> ("SpecAnPlugins.lvlib Out"=w530:refnum<class "SpecAnBase.lvclass">)  [unwired: 11 in]
            n170 = call-dynamic "ConfigureTrigger.vi"("error in (no error)"=w535, "SpecAnBase in"=w530) -> ("error out"=w529:errorcluster, "SpecAnBase out"=w527:refnum<class "SpecAnBase.lvclass">)  [unwired: 8 in]
            n171 = call "CheckOnIdle.vi"("OverwriteClass? (F)"=w526, "error in (no error)"=w529, "ChangeOccured? (F)"=w526, "SpecAnPlugins.lvlib In"=w527) -> ("Error Out"=w528:errorcluster)  [unwired: 6 in, 1 out]
            n172 = call "StatusUpdate.vi"("error in (no error)"=w528, "Status"="Trigger Configured", "Module"=w533) -> ("error out"=w534:errorcluster, "Module"=w532:refnum<class "ModuleAdmin.lvclass">)  [unwired: 7 in]
          }
          frame "InitAcq" {
            n173 = call "SpecAnState.vi"() -> ("State Out"=w543:string)  [unwired: 11 in]
            n174 = Equal?(x=w543, y="Run") -> (x = y?=w540:bool)
            n175 = case shown="False" w540 {
              tunnel: [w545 w551] -> w537
              tunnel: [w544 w552] -> w536
              tunnel: w541 -> [w545 w553]
              tunnel: w538 -> [w544 w554]
              tunnel: w539 -> [_ _]
              frame False {
                n176 = call "SpecAnState.vi"("Set Boolean"=TRUE, "State In"="Start") -> ()  [unwired: 9 in, 1 out]
              }
              frame True {
                n177 = property class="ModuleAdmin.lvclass"(reference=w554, error in=w553) -> (reference out=w552:refnum<class "ModuleAdmin.lvclass">, "Accessors:Module ID"=w549:i32, "Accessors:ModuleName"=w550:string)  [unwired: 1 out]
                n178 = case shown="Default" w549 {
                  selector: w549 -> [w558 _]
                  tunnel: [w556 w559] -> w548
                  tunnel: w550 -> [w557 w559]
                  frame Default {
                    n179 = Format Into String(format string=" %d", initial string=w557, w558) -> (resulting string=w556:string)  [unwired: 1 in, 1 out]
                  }
                  frame ..-1 {
                  }
                }
                n180 = xnode "Error Ring"("parameter 0"=w548) -> ("error out"=w551:errorcluster)
              }
            }
          }
          frame "GetTraceName" {
            n181 = call "anCLASS.vi"() -> ("SpecAnPlugins.lvlib Out"=w576:refnum<class "SpecAnBase.lvclass">)  [unwired: 11 in]
            n182 = call-dynamic "GetTraceName.vi"("error in (no error)"=w580, "SpecAnBase in"=w576) -> ("error out"=w571:errorcluster, "TraceName"=w567:string[], "SpecAnBase out"=w574:refnum<class "SpecAnBase.lvclass">)  [unwired: 7 in]
            n183 = call "anCLASS.vi"("Set? (f)"=TRUE, "SpecAnPlugins.lvlib In"=w574) -> ()  [unwired: 9 in, 1 out]
            n184 = property class="ModuleAdmin.lvclass"(reference=w572, error in=w571) -> (reference out=w569:refnum<class "ModuleAdmin.lvclass">, error out=w570:errorcluster, "Accessors:Module ID"=w568:i32)
            n185 = call "TraceName(s)Broadcast.vi"("error in (no error)"=w570, "TraceName(s)"=w567, "ModuleID"=w568) -> ("error out"=w573:errorcluster)  [unwired: 8 in]
            n186 = call "StatusUpdate.vi"("error in (no error)"=w573, "Status"="Trace(s) Names Extracted", "Module"=w569) -> ("error out"=w579:errorcluster, "Module"=w578:refnum<class "ModuleAdmin.lvclass">)  [unwired: 7 in]
          }
          frame "CloseDevice" {
            w581 = FALSE ("ChangeOccured?")
            n187 = call "anCLASS.vi"() -> ("SpecAnPlugins.lvlib Out"=w583:refnum<class "SpecAnBase.lvclass">)  [unwired: 11 in]
            n188 = call "CheckOnIdle.vi"("OverwriteClass? (F)"=w581, "error in (no error)"=w585, "ChangeOccured? (F)"=w581, "SpecAnPlugins.lvlib In"=w583) -> ("Error Out"=w584:errorcluster, "SpecAnPlugins.lvlib In 2"=w582:refnum<class "SpecAnBase.lvclass">)  [unwired: 6 in]
            n189 = call-dynamic "Close.vi"("error in (no error)"=w584, "SpecAnBase in"=w582) -> ("error out"=w586:errorcluster)  [unwired: 8 in, 1 out]
            n190 = call "StatusUpdate.vi"("error in (no error)"=w586, "Status"="Device Closed", "Module"=w589) -> ("error out"=w590:errorcluster, "Module"=w588:refnum<class "ModuleAdmin.lvclass">)  [unwired: 7 in]
          }
          frame "Abort" {
            n191 = flat-sequence {
              tunnel: w593 -> [w595]
              tunnel: [w595] -> w592
              frame #0 {
                n192 = call "SpecAnState.vi"("Set Boolean"=TRUE, "State In"="Stop") -> ()  [unwired: 9 in, 1 out]
              }
            }
          }
        }
        n193 = call "ErrorHandler.vi"("error in (no error)"=w283, "ModuleAdmin"=w282) -> ("error out"=w284:errorcluster, "ModuleAdmin Out"=w281:refnum<class "ModuleAdmin.lvclass">)  [unwired: 8 in]
      }
      n194 = while {
        tunnel: w40 -> [w54]
        tunnel: [w52] -> w42
        tunnel: w41 -> [w51]
        stop <- w56 stop-if-true
        # "Acquisition Loop"
        n195 = call "SpecAnState.vi"() -> ("State Out"=w55:string)  [unwired: 11 in]
        n196 = case shown="\"Exit\"" w55 {
          tunnel: [FALSE ("Set? (f)") FALSE ("Set? (f)") FALSE ("Set? (f)") FALSE ("Set? (f)") TRUE ("Set? (f)")] -> w56
          tunnel: w54 -> [w59 w68 w81 w104 w118]
          tunnel: [w58 w63 w79 w102 w118] -> w53
          tunnel: w51 -> [w57 w67 w84 w107 w117]
          tunnel: [w57 w66 w83 w106 w117] -> w50
          frame "Idle", Default {
            n197 = flat-sequence {
              tunnel: w59 -> [w61]
              tunnel: [w61] -> w58
              frame #0 {
                n198 = Wait (ms)(milliseconds to wait=u32 50) -> ()  [unwired: 1 out]
              }
            }
          }
          frame "Start" {
            n199 = call "anCLASS.vi"() -> ("SpecAnPlugins.lvlib Out"=w71:refnum<class "SpecAnBase.lvclass">)  [unwired: 11 in]
            n200 = call-dynamic "Initiate.vi"("error in (no error)"=w68, "SpecAnBase in"=w71) -> ("error out"=w69:errorcluster, "SpecAnBase out"=w73:refnum<class "SpecAnBase.lvclass">)  [unwired: 8 in]
            n201 = call "anCLASS.vi"("Set? (f)"=TRUE, "SpecAnPlugins.lvlib In"=w73) -> ()  [unwired: 9 in, 1 out]
            n202 = call "StatusUpdate.vi"("error in (no error)"=w69, "Status"="Acquisition Initiated", "Module"=w67) -> ("error out"=w64:errorcluster, "Module"=w66:refnum<class "ModuleAdmin.lvclass">)  [unwired: 7 in]
            n203 = flat-sequence {
              tunnel: w64 -> [w74]
              tunnel: [w74] -> w63
              frame #0 {
                n204 = call "SpecAnState.vi"("Set Boolean"=TRUE, "State In"="Run") -> ()  [unwired: 9 in, 1 out]
              }
            }
          }
          frame "Run" {
            n205 = call "SpecAnReadorFetch.vi"() -> ("enumFetchorRead"=w77:enum16{"Read", "Fetch"})  [unwired: 11 in]
            n206 = case shown="\"Fetch\"" w77 {
              tunnel: ["Read Trace(s)" ("Status") "Fetched Trace(s)" ("Status")] -> w86
              tunnel: [w88 w94] -> w85
              tunnel: w81 -> [w89 w93]
              frame "Read", Default {
                n207 = call "anCLASS.vi"() -> ("SpecAnPlugins.lvlib Out"=w92:refnum<class "SpecAnBase.lvclass">)  [unwired: 11 in]
                n208 = call-dynamic "Read(Y)Trace.vi"("error in (no error)"=w89, "SpecAnBase in"=w92) -> ("error out"=w88:errorcluster, "SpecAnBase out"=w90:refnum<class "SpecAnBase.lvclass">)  [unwired: 8 in]
                n209 = call "anCLASS.vi"("Set? (f)"=TRUE, "SpecAnPlugins.lvlib In"=w90) -> ()  [unwired: 9 in, 1 out]
              }
              frame "Fetch" {
                n210 = call "anCLASS.vi"() -> ("SpecAnPlugins.lvlib Out"=w96:refnum<class "SpecAnBase.lvclass">)  [unwired: 11 in]
                n211 = call-dynamic "Fetch(Y)Trace.vi"("error in (no error)"=w93, "SpecAnBase in"=w96) -> ("error out"=w94:errorcluster, "SpecAnBase out"=w98:refnum<class "SpecAnBase.lvclass">)  [unwired: 8 in]
                n212 = call "anCLASS.vi"("Set? (f)"=TRUE, "SpecAnPlugins.lvlib In"=w98) -> ()  [unwired: 9 in, 1 out]
              }
            }
            n213 = call "StatusUpdate.vi"("error in (no error)"=w85, "Status"=w86, "Module"=w84) -> ("error out"=w80:errorcluster, "Module"=w83:refnum<class "ModuleAdmin.lvclass">)  [unwired: 7 in]
            n214 = flat-sequence {
              tunnel: w80 -> [w100]
              tunnel: [w100] -> w79
              frame #0 {
                n215 = Unbundle By Name(w100) -> ("status"=w99:bool)
                n216 = call "SpecAnState.vi"("Set Boolean"=w99, "State In"="Stop" ("strngStateIn")) -> ()  [unwired: 9 in, 1 out]
              }
            }
            n217 = Wait (ms)(milliseconds to wait=u32 1000) -> ()  [unwired: 1 out]
          }
          frame "Stop" {
            n218 = call "anCLASS.vi"() -> ("SpecAnPlugins.lvlib Out"=w110:refnum<class "SpecAnBase.lvclass">)  [unwired: 11 in]
            n219 = call-dynamic "Abort.vi"("error in (no error)"=w104, "SpecAnBase in"=w110) -> ("error out"=w108:errorcluster, "SpecAnBase out"=w112:refnum<class "SpecAnBase.lvclass">)  [unwired: 8 in]
            n220 = call "anCLASS.vi"("Set? (f)"=TRUE, "SpecAnPlugins.lvlib In"=w112) -> ()  [unwired: 9 in, 1 out]
            n221 = call "StatusUpdate.vi"("error in (no error)"=w108, "Status"="Acquisiton Aborted", "Module"=w107) -> ("error out"=w103:errorcluster, "Module"=w106:refnum<class "ModuleAdmin.lvclass">)  [unwired: 7 in]
            n222 = flat-sequence {
              tunnel: w103 -> [w113]
              tunnel: [w113] -> w102
              frame #0 {
                n223 = call "SpecAnState.vi"("Set Boolean"=TRUE, "State In"="Idle") -> ()  [unwired: 9 in, 1 out]
              }
            }
          }
          frame "Exit" {
          }
        }
        n224 = call "ErrorHandler.vi"("error in (no error)"=w53, "ModuleAdmin"=w50) -> ("error out"=w52:errorcluster)  [unwired: 8 in, 1 out]
      }
    }
    frame Error {
      n225 = property class="ModuleAdmin.lvclass"(reference=w598) -> (reference out=w602:refnum<class "ModuleAdmin.lvclass">, "Accessors:CloneRegRef"=w601:refnum<data-value>, "Accessors:Module ID"=w600:i32)  [unwired: 1 in, 1 out]
      n226 = call <userlib>:"Remove.vi"("Module ID"=w600, "CloneRegRef"=w601) -> ("error out"=w603:errorcluster)  [unwired: 7 in, 2 out]
      n227 = flat-sequence {
        tunnel: w604 -> [w607]
        tunnel: w603 -> [_]
        tunnel: [w605] -> w597
        frame #0 {
          w606 = T5 2 items=["no dialog", "OK message", "continue or stop message", "OK message + warnings", "continue/stop + warnings"] ("type of dialog (OK msg:1)")
          n228 = call <vilib>:"Simple Error Handler.vi"("type of dialog (OK msg:1)"=w606, "error in (no error)"=w607) -> ("error out"=w605:errorcluster)  [unwired: 3 in, 4 out]
        }
      }
    }
  }
  n229 = Unregister For Events(event registration refnum=w28, error in=w29) -> (error out=w27:errorcluster)
  n230 = call "ObtainQueue.vi"("error in (no error)"=w3, "create if not found? (f)"=FALSE ("create if not found? (T)"), "ModuleAdmin"=w4) -> ("error out"=w12:errorcluster, "queue out"=w20:refnum<queue>, "ModuleAdmin Out"=w8:refnum<class "ModuleAdmin.lvclass">)  [unwired: 6 in]
  n231 = Release Queue(queue=w20, force destroy? (F)=FALSE, error in (no error)=w12) -> (error out=w10:errorcluster)  [unwired: 2 out]
  n232 = call "DestroyClone.vi"("error in (no error)"=w10, "Exit via Stop Module Req?"=w6, "Wait for Module to stop?"=w7, "ModuleAdmin"=w8) -> ("error out"=w9:errorcluster, "External Launch"=w5:bool)  [unwired: 5 in, 1 out]
  n233 = Merge Errors(w27, w9, w1) -> (w11:errorcluster)
  n234 = case shown="True" w5 {
    tunnel: w11 -> [w608 w611]
    tunnel: [w608 w609] -> w2
    frame False {
    }
    frame True {
      n235 = control-ref of="This VI"() -> (w610:refnum<vi>)
      n236 = case shown="No Error" w611 {
        selector: w611 -> [w615 w617]
        tunnel: w610 -> [w616 w618]
        tunnel: [w612 w617] -> w609
        frame No Error {
          n237 = invoke class="VI" method="FP.Close"(reference=w616, error in=w615) -> (reference out=w613:refnum<vi>, error out=w614:errorcluster)  [unwired: 1 in, 1 out]
          n238 = Close Reference(reference=w613, error in (no error)=w614) -> (error out=w612:errorcluster)
        }
        frame Error {
          n239 = invoke class="VI" method="FP.Open"(reference=w618, "Activate"=TRUE ("Activate?")) -> ()  [unwired: 3 in, 5 out]
        }
      }
    }
  }
  "error out" <- w2
